vi "Write Status Str Refnum.vi"(8 "error in (no error)":errorcluster, 10 "Status Str Refnum":refnum<vi>, 11 "Tesla Factory Tester in":refnum<class "Tesla Factory Tester.lvclass">) -> (0 "error out":errorcluster, 3 "Tesla Factory Tester out":refnum<class "Tesla Factory Tester.lvclass">)   [LabVIEW 2013, in "Tesla Factory Tester.lvlib" / "Tesla Factory Tester.lvclass"]
uses:
  Tesla Factory Tester.lvclass
  Tesla Factory Tester.lvclass/Tesla Factory Tester.ctl
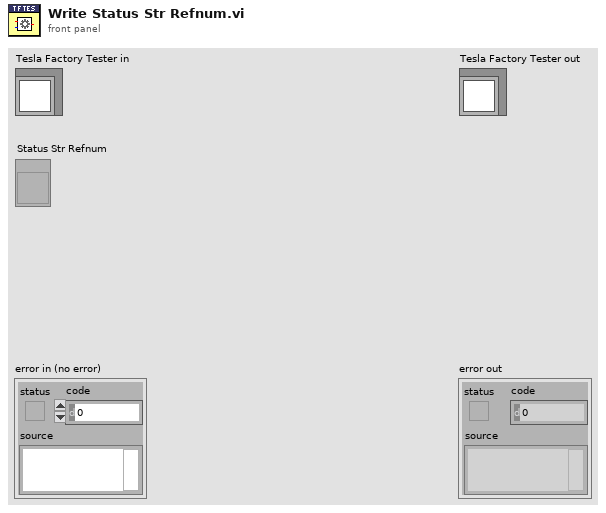
[diagram p1: front panel]
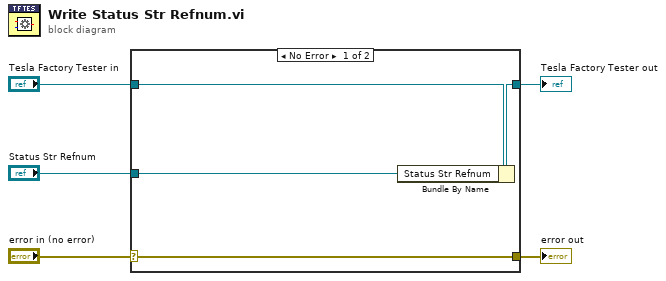
[diagram p0: block diagram]
diagram:
  n1 = case shown="No Error" "error in (no error)" {
    selector: "error in (no error)" -> [w9 w10]
    tunnel: [w9 w10] -> w4
    tunnel: [w7 w11] -> w2
    tunnel: "Tesla Factory Tester in" -> [w8 w11]
    tunnel: "Status Str Refnum" -> [w6 _]
    frame No Error {
      n2 = Bundle By Name(cluster=w8, "Status Str Refnum"=w6) -> (w7:refnum<class "Tesla Factory Tester.lvclass">)
    }
    frame Error {
    }
  }
  "error out" <- w4
  "Tesla Factory Tester out" <- w2
